vi "Core Actor - CLOSE - External Queues_Notifiers.vi"(8 "error in (no error)":errorcluster, 11 "Interface_Class in":refnum<class "SW_Interface_Class.lvclass">) -> (0 "error out":errorcluster, 3 "Interface_Class out":refnum<class "SW_Interface_Class.lvclass">)   [LabVIEW 2023, in "SW_Interface_Actor.lvlib" / "SW_Interface_Class.lvclass"]
uses:
  SW_Interface_Class.lvclass
  SW_Interface_Class.lvclass/SW_Interface_Class.ctl
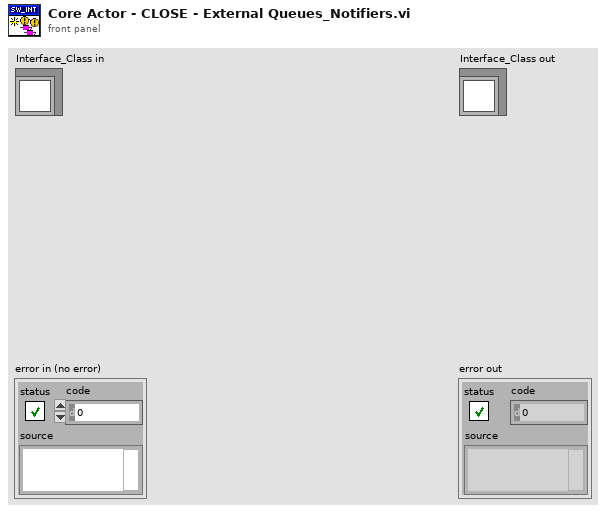
[diagram p1: front panel]
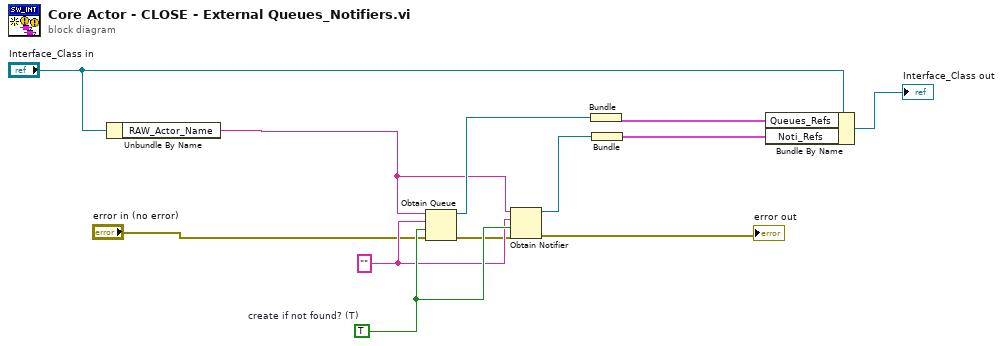
[diagram p0: block diagram]
diagram:
  w12 = TRUE  # create if not found? (T)
  w11 = ""
  n1 = Unbundle By Name("Interface_Class in") -> ("RAW_Actor_Name"=w4:string)
  n2 = Obtain Queue(name (unnamed)=w4, element data type=w11, create if not found? (T)=w12, error in (no error)="error in (no error)") -> (queue out=w9:refnum<queue>, error out=w10:errorcluster)  [unwired: 1 in, 1 out]
  n3 = Obtain Notifier(name (unnamed)=w4, notification data type=w11, create if not found? (T)=w12, error in (no error)=w10) -> (notifier out=w8:refnum<notifier>, error out=→"error out":errorcluster)  [unwired: 1 out]
  n4 = Bundle("queue out"=w9) -> (w3:cluster{"queue out":refnum<queue>})  [unwired: 1 in]
  n5 = Bundle("notifier out"=w8) -> (w2:cluster{"notifier out":refnum<notifier>})  [unwired: 1 in]
  n6 = Bundle By Name(cluster="Interface_Class in", "Queues_Refs"=w3, "Noti_Refs"=w2) -> (→"Interface_Class out":refnum<class "SW_Interface_Class.lvclass">)
